vi "Finish.vi"   [LabVIEW 2012]
doc: "This VI is called just before exiting. It is expected to close I/O refnum, save collected data, etc."
uses:
  <vilib>/Rock Robotics/WPI/Compressor/WPI_CompressorGetSetRefNum.vi
  <vilib>/Rock Robotics/WPI/Joystick/WPI_JoystickGetSetRefNum.vi
  <vilib>/Rock Robotics/WPI/RobotDrive/WPI_RobotDriveGetSetRefNum.vi
types:
  T1 = typedef "WPI_MotorControlDeviceRef.ctl" = cluster{"DeviceStatus":errorcluster, "Type":enum16{"PWM", "CAN"}, "PWM":cluster{"Digital Module":T2, "PWM Channel":T3, "DeadBand":T4}, "CAN":cluster{"Device Number":u8, "Control Mode":T5, "Semaphore":T6, "Max Vout":dbl}, "Invert":bool, "TransformRef":T7, "InvTransformRef":T7}
  T2 = typedef "FPGA_TypedefDigitalModule.ctl" = enum16{"Digital Module 1", "Digital Module 2"}
  T3 = typedef "FPGA_DIOPWMChannel.ctl" = enum8{"PWM 1", "PWM 2", "PWM 3", "PWM 4", "PWM 5", "PWM 6", "PWM 7", "PWM 8", "PWM 9", "PWM 10", "Invalid"}
  T4 = typedef "WPI_PWMDeadband.ctl" = cluster{"Name":string, "maxPositivePwm":i32, "minPositivePwm":i32, "centerPwm":i32, "maxNegativePwm":i32, "minNegativePwm":i32, "angularRange":u16}
  T5 = typedef "WPI_CANJaguar_ControlMode.ctl" = enum8{"Percent VBus", "Current", "Speed", "Position", "Voltage"}
  T6 = typedef "Semaphore RefNum" = refnum<k1>
  T7 = typedef "WPI_PWMTransform_ConPane.ctl" = refnum<vi>
  T8 = typedef "WPI_JoystickDevRef.ctl" = cluster{"Device":T9}
  T9 = typedef "WPI_JoystickDeviceEnum.ctl" = enum16{"USB 1", "USB 2", "USB 3", "USB 4", "Kinect 1", "Kinect 2"}
  T10 = typedef "WPI_RelayDevRef.ctl" = cluster{"DevStatus":errorcluster, "Relay Channel":T11, "Digital Module":T2, "Relay Direction":T12}
  T11 = typedef "FPGA_DIORelayChannel.ctl" = enum8{"Relay 1", "Relay 2", "Relay 3", "Relay 4", "Relay 5", "Relay 6", "Relay 7", "Relay 8", "Invalid"}
  T12 = typedef "WPI_RelayDirection.ctl" = enum16{"Both directions", "Forward only", "Reverse only"}
  T13 = typedef "WPI_DigitalInputDevRef.ctl" = cluster{"DevStatus":errorcluster, "DIO Channel":T14, "Digital Module":T2}
  T14 = typedef "FPGA_DIOChannel.ctl" = enum8{"DIO 1", "DIO 2", "DIO 3", "DIO 4", "DIO 5", "DIO 6", "DIO 7", "DIO 8", "DIO 9", "DIO 10", "DIO 11", "DIO 12", "DIO 13", "DIO 14", "Invalid"}
  T15 = typedef "WPI_ServoDeviceRef.ctl" = cluster{"DeviceStatus":errorcluster, "Digital Module":T2, "PWM Channel":T3, "DeadBand":T4}
  T16 = typedef "WPI_AnalogChannelDevRef.ctl" = cluster{"DevStatus":errorcluster, "Analog Module":T17, "Analog Channel":T18}
  T17 = typedef "FPGA_TypedefAnalogModule.ctl" = enum16{"Analog Module 1", "Analog Module 2"}
  T18 = typedef "FPGA_AIChannel.ctl" = enum8{"AI 1", "AI 2", "AI 3", "AI 4", "AI 5", "AI 6", "AI 7", "AI 8", "Invalid"}
  T19 = typedef "WPI_CompressorDevRef.ctl" = cluster{"DevStatus":errorcluster, "DigitalInputDevRef":T13, "RelayDevRef":T10}
  T20 = typedef "WPI_CounterDevRef.ctl" = cluster{"DevStatus":errorcluster, "CntIndex":T21}
  T21 = typedef "FPGA_CounterCtrSystemIndex.ctl" = enum8{"Ctr 0", "Ctr 1", "Ctr 2", "Ctr 3", "Ctr 4", "Ctr 5", "Ctr 6", "Ctr 7", "Invalid"}
  T22 = typedef "WPI_SolenoidDevRef.ctl" = cluster{"DevStatus":errorcluster, "Solenoid Module":T23, "Forward Solenoid Channel":T24, "Reverse Solenoid Channel":T24}
  T23 = typedef "FPGA_TypedefSolenoidModule.ctl" = enum16{"Solenoid Module 1", "Solenoid Module 2"}
  T24 = typedef "WPI_SolenoidChannel.ctl" = enum8{"Solenoid 1", "Solenoid 2", "Solenoid 3", "Solenoid 4", "Solenoid 5", "Solenoid 6", "Solenoid 7", "Solenoid 8", "Invalid"}
  T25 = typedef "WPI_RobotDriveDevRef.ctl" = cluster{"DevStatus":errorcluster, "Motors[]":T1[], "Square Inputs":bool, "Max Output":dbl, "Isochronous":bool}
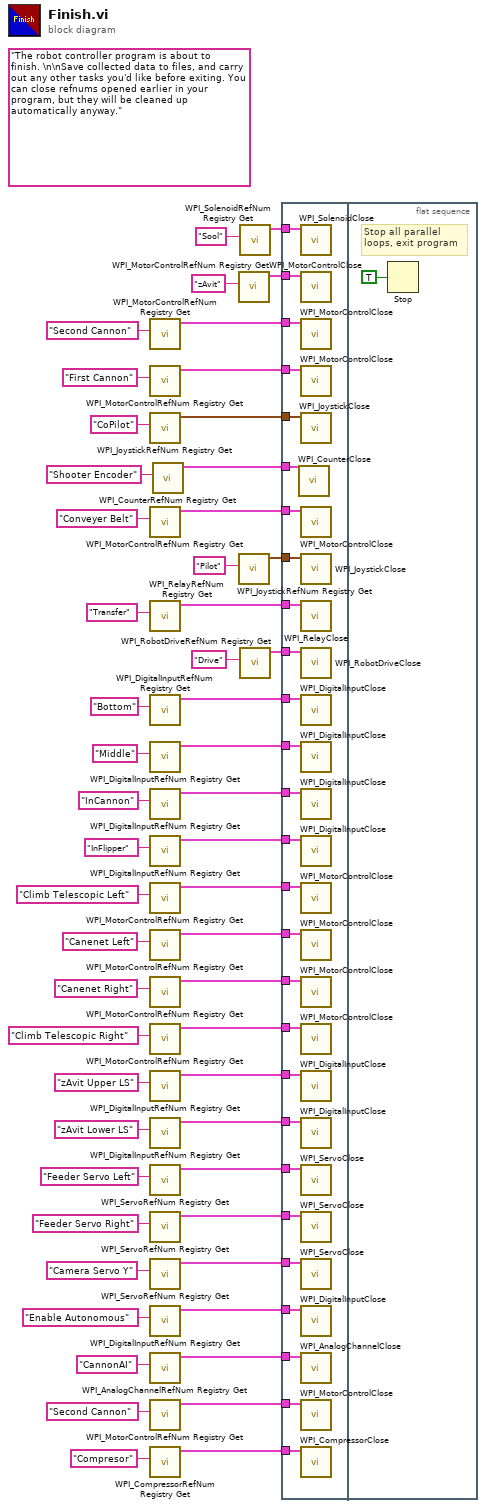
[diagram p0: block diagram]
diagram:
  (unwired) "The robot controller program is about to finish. \n\nSave collected data to files, and carry out any other tasks you'd like before exiting. You can close refnums opened earlier in your program, but they will be cleaned up automatically anyway."
  n1 = call <vilib>:"WPI_MotorControlRefNum Registry Get.vi"("refnum name"="Second Cannon") -> ("MotorControlDevRef"=w47:T1)  [unwired: 9 in, 1 out]
  n2 = call <vilib>:"WPI_MotorControlRefNum Registry Get.vi"("refnum name"="First Cannon") -> ("MotorControlDevRef"=w46:T1)  [unwired: 9 in, 1 out]
  n3 = call <vilib>:"WPI_JoystickRefNum Registry Get.vi"("refnum name"="CoPilot") -> ("JoystickDevRef"=w44:T8)  [unwired: 9 in, 1 out]
  n4 = call <vilib>:"WPI_MotorControlRefNum Registry Get.vi"("refnum name"="Conveyer Belt") -> ("MotorControlDevRef"=w41:T1)  [unwired: 9 in, 1 out]
  n5 = call <vilib>:"WPI_RelayRefNum Registry Get.vi"("refnum name"="Transfer") -> ("RelayDevRef"=w39:T10)  [unwired: 9 in, 1 out]
  n6 = call <vilib>:"WPI_DigitalInputRefNum Registry Get.vi"("refnum name"="Bottom") -> ("DigitalInputDevRef"=w34:T13)  [unwired: 9 in, 1 out]
  n7 = call <vilib>:"WPI_DigitalInputRefNum Registry Get.vi"("refnum name"="Middle") -> ("DigitalInputDevRef"=w33:T13)  [unwired: 9 in, 1 out]
  n8 = call <vilib>:"WPI_DigitalInputRefNum Registry Get.vi"("refnum name"="InCannon") -> ("DigitalInputDevRef"=w32:T13)  [unwired: 9 in, 1 out]
  n9 = call <vilib>:"WPI_DigitalInputRefNum Registry Get.vi"("refnum name"="InFlipper") -> ("DigitalInputDevRef"=w31:T13)  [unwired: 9 in, 1 out]
  n10 = call <vilib>:"WPI_MotorControlRefNum Registry Get.vi"("refnum name"="Climb Telescopic Left") -> ("MotorControlDevRef"=w26:T1)  [unwired: 9 in, 1 out]
  n11 = call <vilib>:"WPI_MotorControlRefNum Registry Get.vi"("refnum name"="Canenet Left") -> ("MotorControlDevRef"=w25:T1)  [unwired: 9 in, 1 out]
  n12 = call <vilib>:"WPI_MotorControlRefNum Registry Get.vi"("refnum name"="Canenet Right") -> ("MotorControlDevRef"=w24:T1)  [unwired: 9 in, 1 out]
  n13 = call <vilib>:"WPI_MotorControlRefNum Registry Get.vi"("refnum name"="Climb Telescopic Right") -> ("MotorControlDevRef"=w23:T1)  [unwired: 9 in, 1 out]
  n14 = call <vilib>:"WPI_DigitalInputRefNum Registry Get.vi"("refnum name"="zAvit Upper LS") -> ("DigitalInputDevRef"=w20:T13)  [unwired: 9 in, 1 out]
  n15 = call <vilib>:"WPI_DigitalInputRefNum Registry Get.vi"("refnum name"="zAvit Lower LS") -> ("DigitalInputDevRef"=w19:T13)  [unwired: 9 in, 1 out]
  n16 = call <vilib>:"WPI_ServoRefNum Registry Get.vi"("refnum name"="Feeder Servo Left") -> ("ServoDeviceRef"=w16:T15)  [unwired: 9 in, 1 out]
  n17 = call <vilib>:"WPI_ServoRefNum Registry Get.vi"("refnum name"="Feeder Servo Right") -> ("ServoDeviceRef"=w15:T15)  [unwired: 9 in, 1 out]
  n18 = call <vilib>:"WPI_ServoRefNum Registry Get.vi"("refnum name"="Camera Servo Y") -> ("ServoDeviceRef"=w13:T15)  [unwired: 9 in, 1 out]
  n19 = call <vilib>:"WPI_DigitalInputRefNum Registry Get.vi"("refnum name"="Enable Autonomous") -> ("DigitalInputDevRef"=w11:T13)  [unwired: 9 in, 1 out]
  n20 = call <vilib>:"WPI_AnalogChannelRefNum Registry Get.vi"("refnum name"="CannonAI") -> ("AIDeviceRef"=w9:T16)  [unwired: 9 in, 1 out]
  n21 = call <vilib>:"WPI_MotorControlRefNum Registry Get.vi"("refnum name"="Second Cannon") -> ("MotorControlDevRef"=w7:T1)  [unwired: 9 in, 1 out]
  n22 = call <vilib>:"WPI_CompressorRefNum Registry Get.vi"("refnum name"="Compresor") -> ("CompressorDevRef"=w4:T19)  [unwired: 9 in, 1 out]
  n23 = call <vilib>:"WPI_CounterRefNum Registry Get.vi"("refnum name"="Shooter Encoder") -> ("CounterDevRef"=w1:T20)  [unwired: 9 in, 1 out]
  n24 = call <vilib>:"WPI_MotorControlRefNum Registry Get.vi"("refnum name"="zAvit") -> ("MotorControlDevRef"=w51:T1)  [unwired: 9 in, 1 out]
  n25 = call <vilib>:"WPI_JoystickRefNum Registry Get.vi"("refnum name"="Pilot") -> ("JoystickDevRef"=w53:T8)  [unwired: 1 in, 9 out]
  n26 = call <vilib>:"WPI_SolenoidRefNum Registry Get.vi"("refnum name"="Sool") -> ("SolenoidDevRef"=w3:T22)  [unwired: 9 in, 1 out]
  n27 = call <vilib>:"WPI_RobotDriveRefNum Registry Get.vi"("refnum name"="Drive") -> ("RobotDriveDevRef"=w54:T25)  [unwired: 1 in, 9 out]
  n28 = flat-sequence {
    tunnel: w54 -> [w81]
    tunnel: w53 -> [w80]
    tunnel: w51 -> [w79]
    tunnel: w47 -> [w78]
    tunnel: w46 -> [w77]
    tunnel: w44 -> [w76]
    tunnel: w41 -> [w75]
    tunnel: w39 -> [w74]
    tunnel: w34 -> [w73]
    tunnel: w33 -> [w72]
    tunnel: w32 -> [w71]
    tunnel: w31 -> [w70]
    tunnel: w26 -> [w69]
    tunnel: w25 -> [w68]
    tunnel: w24 -> [w67]
    tunnel: w23 -> [w66]
    tunnel: w20 -> [w65]
    tunnel: w19 -> [w64]
    tunnel: w16 -> [w63]
    tunnel: w15 -> [w62]
    tunnel: w13 -> [w61]
    tunnel: w11 -> [w60]
    tunnel: w9 -> [w59]
    tunnel: w7 -> [w58]
    tunnel: w4 -> [w57]
    tunnel: w3 -> [w56]
    tunnel: w1 -> [w55]
    frame #0 {
      n29 = call <vilib>:"WPI_CounterClose.vi"("CounterDevRef"=w55) -> ()  [unwired: 10 in, 1 out]
      n30 = call <vilib>:"WPI_SolenoidClose.vi"("SolenoidDevRef"=w56) -> ()  [unwired: 10 in, 1 out]
      n31 = call <vilib>:"WPI_MotorControlClose.vi"("MotorControlDevRef"=w79) -> ()  [unwired: 10 in, 1 out]
      n32 = call <vilib>:"WPI_MotorControlClose.vi"("MotorControlDevRef"=w78) -> ()  [unwired: 10 in, 1 out]
      n33 = call <vilib>:"WPI_MotorControlClose.vi"("MotorControlDevRef"=w77) -> ()  [unwired: 10 in, 1 out]
      n34 = call <vilib>:"WPI_JoystickClose.vi"("JoystickDevRef"=w76) -> ()  [unwired: 11 out]
      n35 = call <vilib>:"WPI_MotorControlClose.vi"("MotorControlDevRef"=w75) -> ()  [unwired: 10 in, 1 out]
      n36 = call <vilib>:"WPI_JoystickClose.vi"("JoystickDevRef"=w80) -> ()  [unwired: 11 out]
      n37 = call <vilib>:"WPI_RelayClose.vi"("RelayDevRef"=w74) -> ()  [unwired: 10 in, 1 out]
      n38 = call <vilib>:"WPI_RobotDriveClose.vi"("RobotDriveDevRef"=w81) -> ()  [unwired: 1 in, 10 out]
      n39 = call <vilib>:"WPI_DigitalInputClose.vi"("DigitalInputDevRef"=w73) -> ()  [unwired: 10 in, 1 out]
      n40 = call <vilib>:"WPI_DigitalInputClose.vi"("DigitalInputDevRef"=w72) -> ()  [unwired: 10 in, 1 out]
      n41 = call <vilib>:"WPI_DigitalInputClose.vi"("DigitalInputDevRef"=w71) -> ()  [unwired: 10 in, 1 out]
      n42 = call <vilib>:"WPI_DigitalInputClose.vi"("DigitalInputDevRef"=w70) -> ()  [unwired: 10 in, 1 out]
      n43 = call <vilib>:"WPI_MotorControlClose.vi"("MotorControlDevRef"=w69) -> ()  [unwired: 10 in, 1 out]
      n44 = call <vilib>:"WPI_MotorControlClose.vi"("MotorControlDevRef"=w68) -> ()  [unwired: 10 in, 1 out]
      n45 = call <vilib>:"WPI_MotorControlClose.vi"("MotorControlDevRef"=w67) -> ()  [unwired: 10 in, 1 out]
      n46 = call <vilib>:"WPI_MotorControlClose.vi"("MotorControlDevRef"=w66) -> ()  [unwired: 10 in, 1 out]
      n47 = call <vilib>:"WPI_DigitalInputClose.vi"("DigitalInputDevRef"=w65) -> ()  [unwired: 10 in, 1 out]
      n48 = call <vilib>:"WPI_DigitalInputClose.vi"("DigitalInputDevRef"=w64) -> ()  [unwired: 10 in, 1 out]
      n49 = call <vilib>:"WPI_ServoClose.vi"("MotorControlDevRef"=w63) -> ()  [unwired: 10 in, 1 out]
      n50 = call <vilib>:"WPI_ServoClose.vi"("MotorControlDevRef"=w62) -> ()  [unwired: 10 in, 1 out]
      n51 = call <vilib>:"WPI_ServoClose.vi"("MotorControlDevRef"=w61) -> ()  [unwired: 10 in, 1 out]
      n52 = call <vilib>:"WPI_DigitalInputClose.vi"("DigitalInputDevRef"=w60) -> ()  [unwired: 10 in, 1 out]
      n53 = call <vilib>:"WPI_AnalogChannelClose.vi"("AIDeviceRef"=w59) -> ()  [unwired: 10 in, 1 out]
      n54 = call <vilib>:"WPI_MotorControlClose.vi"("MotorControlDevRef"=w58) -> ()  [unwired: 10 in, 1 out]
      n55 = call <vilib>:"WPI_CompressorClose.vi"("CompressorDevRef"=w57) -> ()  [unwired: 10 in, 1 out]
    }
    frame #1 {
      # "Stop all parallel\nloops, exit program"
      n56 = Stop(stop? (T)=TRUE ("Quit")) -> ()
    }
  }
